vi "create Direction.vi"(8 "error in (no error)":errorcluster, 9 "Player":refnum<class "Player.lvclass">, 10 "Direction":T1, 11 "Direction in":refnum<class "Direction.lvclass">) -> (0 "error out":errorcluster, 3 "Direction out":refnum<class "Direction.lvclass">)   [LabVIEW 2019, in "Direction.lvclass"]
uses:
  Direction.lvclass
  Direction STYP.ctl
  Player/Player.lvclass
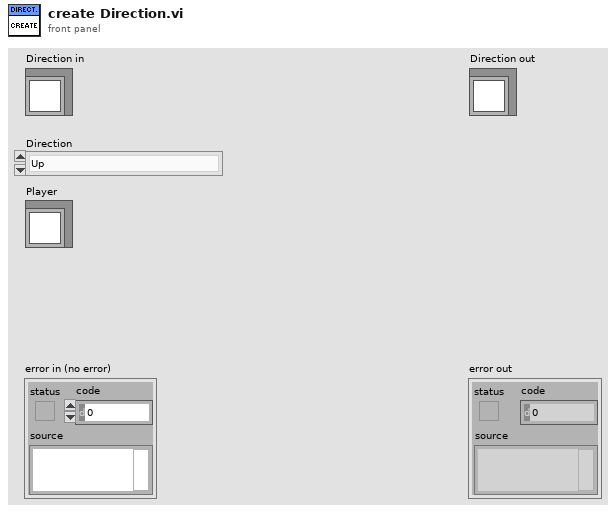
[diagram p1: front panel]
types:
  T1 = typedef "Direction STYP.ctl" = enum16{"Up", "Down", "Left", "Right"}
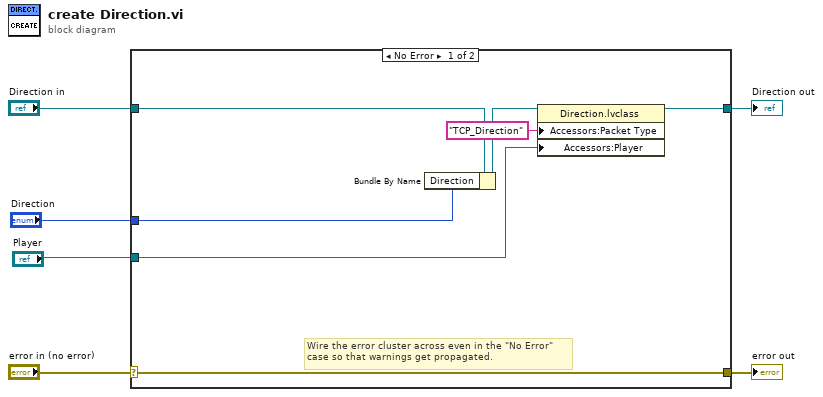
[diagram p0: block diagram]
diagram:
  n1 = case shown="No Error" "error in (no error)" {
    selector: "error in (no error)" -> [w13 w15]
    tunnel: [w13 w15] -> w5
    tunnel: [w9 w14] -> w3
    tunnel: "Direction in" -> [w10 w14]
    tunnel: "Direction" -> [w11 _]
    tunnel: "Player" -> [w8 _]
    frame No Error {
      # "Wire the error cluster across even in the \"No Error\"\ncase so that warnings get propagated."
      n2 = Bundle By Name(cluster=w10, "Direction"=w11) -> (w12:refnum<class "Direction.lvclass">)
      n3 = property class="Direction.lvclass"(reference=w12, "Accessors:Packet Type"="TCP_Direction" ("Packet Type"), "Accessors:Player"=w8) -> (reference out=w9:refnum<class "Direction.lvclass">)  [unwired: 1 in, 1 out]
    }
    frame Error {
    }
  }
  "error out" <- w5
  "Direction out" <- w3
